vi "NF87XX.open Services.vi"(0 "i ref in":refnum<vi>, 5 "error in (no error)":errorcluster) -> (14 "i ref out":refnum<vi>, 19 "error out":errorcluster)   [LabVIEW 2014, in "NF87XX.lvlib"]
doc: "In this VI several DIM services are opened."
uses:
  NF87XX.lvlib
  CSPhelix/PH_StatusHandler/PH_StatusHandler.Status.ctl
  CSPhelix/PH_StatusHandler/PH_StatusHandler.lvlib
  CSPhelix/PH_Common/PH_Common.lvlib
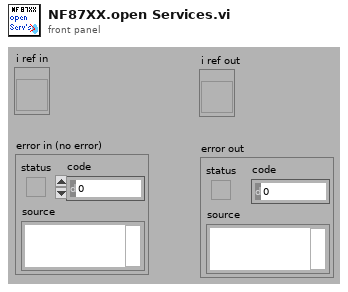
[diagram p1: front panel]
types:
  T1 = typedef "NF87XX.lvlib/NF87XX.i attribute.ctl" = cluster{"Con Settings":T2, "Drivers":T3[], "Status":cluster{"Service ID":i32, "Status":T6}, "Joystick available":bool, "VISA Resource":string}
  T2 = typedef "NewFocusPico - Driver np.lvlib/VISA & TCPIP Control.ctl" = cluster{"VISA or TCP/IP":bool, "Init Connection":bool, "Close Connection":bool, "Resource Name":refnum<visa-resource-name>, "hostname":string, "connection ID":refnum<k5>}
  T3 = typedef "NF87XX.lvlib/NF87XX.driver Settings.ctl" = cluster{"Name":string, "Driver Type":T4, "Pico Parameter type":T5, "Acceleration [Steps/s²]":cluster{"Motor 0":dbl, "Motor 1":dbl, "Motor 2":dbl}, "Start Velocity [Steps/s]":cluster{"Motor 0":dbl, "Motor 1":dbl, "Motor 2":dbl}, "Velocity [Steps/s]":cluster{"Motor 0":dbl, "Motor 1":dbl, "Motor 2":dbl}, "axis channel":i32, "Position":i32, "Position Service ID":i32}
  T4 = typedef "NF87XX.lvlib/NF87XX.driver Type.ctl" = enum16{"not defined", "3-ch open loop drv", "1-ch closed loop drv"}
  T5 = typedef "NewFocusPico - Driver np.lvlib/Pico Parameters.ctl" = cluster{"Pico Type":enum16{"Open-Loop Pico", "Close-Loop Pico", "Pico Ultra"}, "Acceleration (steps/sec^2)":string, "Velocity ( Hz)":string, "Driver":string, "Motor":string, "Channel":string, "Process Step":string}
  T6 = typedef "PH_StatusHandler.lvlib/PH_StatusHandler.Status.ctl" = i16
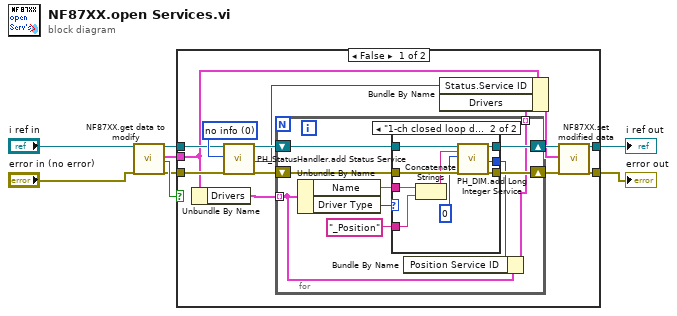
[diagram p0: block diagram]
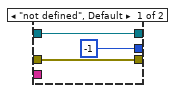
[diagram p2: hidden frame]
diagram:
  n1 = call "NF87XX.get data to modify.vi"("i ref in"="i ref in", "error in (no error)"="error in (no error)") -> ("i ref out"=w2:refnum<vi>, "i attribute"=w6:T1, "timed out"=w5:bool, "error out"=w4:errorcluster)  [unwired: 14 in]
  n2 = case shown="False" w5 {
    tunnel: [w19 w45] -> w8
    tunnel: w2 -> [w17 w46]
    tunnel: w4 -> [w16 w45]
    tunnel: [w14 w46] -> w7
    tunnel: w6 -> [w11 _]
    frame False {
      w22 = T6 0 items=["no info", "off/false/out", "on/true/in", "Failure", "Alarm", "Status 1", "Status 2", "Status 3"] ("Status")
      n3 = Unbundle By Name(w11) -> ("Drivers"=w10:T3[])
      n4 = call "PH_StatusHandler.add Status Service.vi"("i ref in"=w17, "Status"=w22, "error in (no error)"=w16) -> ("i ref out"=w20:refnum<vi>, "Service ID Status"=w12:i32, "error out"=w21:errorcluster)  [unwired: 14 in]
      n5 = for {
        shift-right: [w29] -> w15
        shift-left: w20 -> [w31]
        shift-right: [w30] -> w18
        shift-left: w21 -> [w32]
        tunnel: w10 -> [w25] mode=indexing
        tunnel: [w23] -> w9 mode=indexing
        n6 = Unbundle By Name(w25) -> ("Name"=w27:string, "Driver Type"=w28:T4)
        n7 = case shown="\"1-ch closed loop drv\"" w28 {
          tunnel: w32 -> [w34 w44]
          tunnel: w31 -> [w35 w43]
          tunnel: [w34 w42] -> w30
          tunnel: [w35 w41] -> w29
          tunnel: [-1 ("Service ID") w40] -> w24
          tunnel: w27 -> [_ w39]
          tunnel: "_Position" -> [_ w38]
          frame "not defined", Default {
          }
          frame "1-ch closed loop drv" {
            n8 = Concatenate Strings(w39, w38) -> (w37:string)
            n9 = call "PH_DIM.add Long Integer Service.vi"("i ref in"=w43, "Service Name"=w37, "Number"=0, "error in (no error)"=w44) -> ("i ref out"=w41:refnum<vi>, "Service ID"=w40:i32, "error out"=w42:errorcluster)  [unwired: 13 in]
          }
        }
        n10 = Bundle By Name(cluster=w25, "Position Service ID"=w24) -> (w23:T3)
      }
      n11 = Bundle By Name(cluster=w11, "Status.Service ID"=w12, "Drivers"=w9) -> (w13:T1)
      n12 = call "NF87XX.set modified data.vi"("i ref in"=w15, "i attribute"=w13, "error in (no error)"=w18) -> ("i ref out"=w14:refnum<vi>, "error out"=w19:errorcluster)  [unwired: 15 in]
    }
    frame True {
    }
  }
  "error out" <- w8
  "i ref out" <- w7
